vi "Configure Mark.vi"(8 "error in (no error)":errorcluster, 9 "Operation (0: Create Mark)":i32(ring) items=["Create Mark", "Delete Mark", "Next Mark", "Previous Mark"], 10 "Channel (0: Channel 1)":i32(ring) items=["Channel 1", "Channel 2", "Channel 3", "Channel 4", "Math", "Bus 1", "Bus 2", "Bus 3", "Bus 4", "Reference 1", "Reference 2", "Reference 3", "Reference 4", "Column", "Digital"], 11 "VISA resource name":refnum<visa-resource-name>) -> (0 "error out":errorcluster, 3 "VISA resource name out":refnum<visa-resource-name>)   [LabVIEW 2009, in "Tektronix DPO MSO 2000 4000 Series.lvlib"]
doc: "Configures a mark on a specified waveform or all waveforms according to <B>Operation</B>."
uses:
  <instrlib>/Tektronix DPO MSO 2000 4000 Series/Tektronix DPO MSO 2000 4000 Series.lvlib
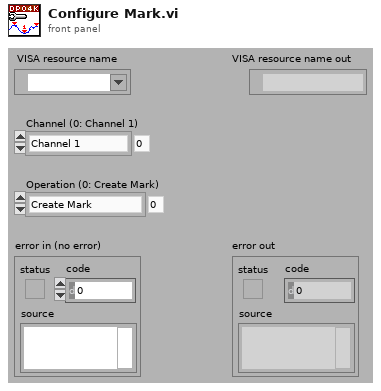
[diagram p1: front panel]
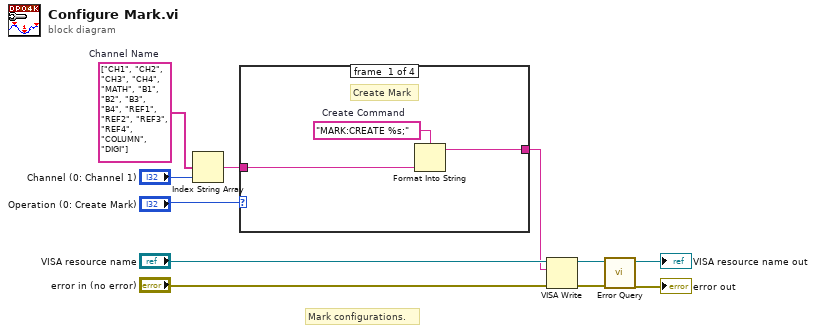
[diagram p0: block diagram]
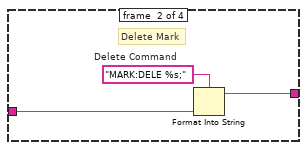
[diagram p2: hidden frame]
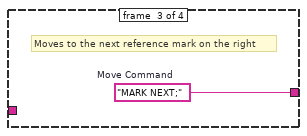
[diagram p3: hidden frame]
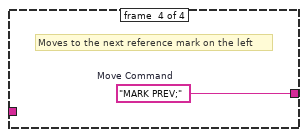
[diagram p4: hidden frame]
diagram:
  w3 = string[] ["CH1", "CH2", "CH3", "CH4", "MATH", "B1", "B2", "B3", "B4", "REF1", "REF2", "REF3", "REF4", "COLUMN", "DIGI"]  # Channel Name
  # "Mark configurations."
  n1 = Index String Array(1:"Channel (0: Channel 1)", 2:w3) -> (0:w2:string)  [unwired: 1 in]
  n2 = case shown="0, Default" "Operation (0: Create Mark)" {
    tunnel: w2 -> [w13 w16 _ _]
    tunnel: [w12 w15 w18 w19] -> w1
    frame #0 {
      w14 = "MARK:CREATE %s;"  # Create Command
      # "Create Mark"
      n3 = Format Into String(format string=w14, w13) -> (resulting string=w12:string)  [unwired: 2 in, 1 out]
    }
    frame #1 {
      w17 = "MARK:DELE %s;"  # Delete Command
      # "Delete Mark"
      n4 = Format Into String(format string=w17, w16) -> (resulting string=w15:string)  [unwired: 2 in, 1 out]
    }
    frame #2 {
      w18 = "MARK NEXT;"  # Move Command
      # "Moves to the next reference mark on the right"
    }
    frame #3 {
      w19 = "MARK PREV;"  # Move Command
      # "Moves to the next reference mark on the left"
    }
  }
  n5 = VISA Write(VISA resource name="VISA resource name", write buffer=w1, error in (no error)="error in (no error)") -> (VISA resource name out=w9:refnum<visa-resource-name>, error out=w8:errorcluster)  [unwired: 1 out]
  n6 = call <instrlib>:"Error Query.vi"("error in (no error)"=w8, "VISA resource name"=w9) -> ("error out"=→"error out":errorcluster, "VISA resource name out"=→"VISA resource name out":refnum<visa-resource-name>)  [unwired: 6 in, 2 out]
